vi "Respond.vi"(6 "String buffer in":string, 7 "String":string, 8 "error in (no error)":errorcluster, 9 "Return Request in":T1, 10 "Boolean in":bool, 11 "String 2":string) -> (0 "error out":errorcluster, 2 "String buffer out":string, 3 "Boolean out":bool)   [LabVIEW 2017, in "SSH.lvlib"]
uses:
  SSH.lvlib
  Return Request Configuration.ctl
  Response Configuration.ctl
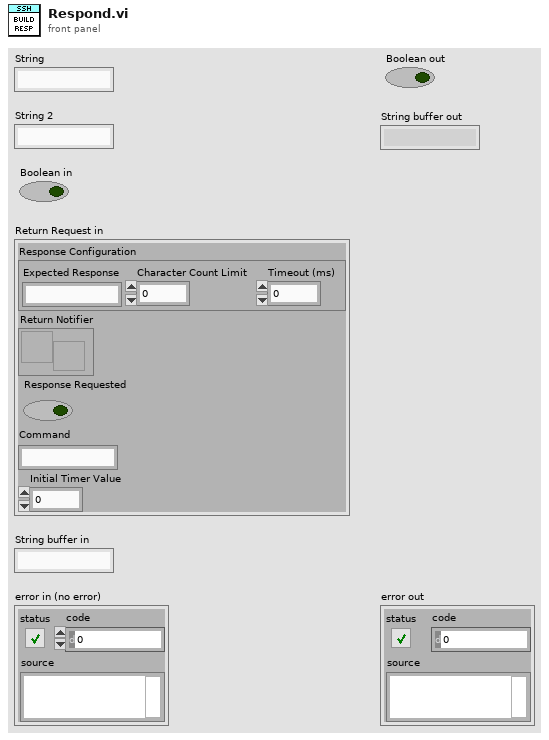
[diagram p1: front panel]
types:
  T1 = typedef "SSH.lvlib/Return Request Configuration.ctl" = cluster{"Response Configuration":T2, "Return Notifier":refnum<notifier>, "Response Requested":bool, "Command":string, "Initial Timer Value":u32}
  T2 = typedef "SSH.lvlib/Response Configuration.ctl" = cluster{"Expected Response":string, "Character Count Limit":i32, "Timeout (ms)":u32}
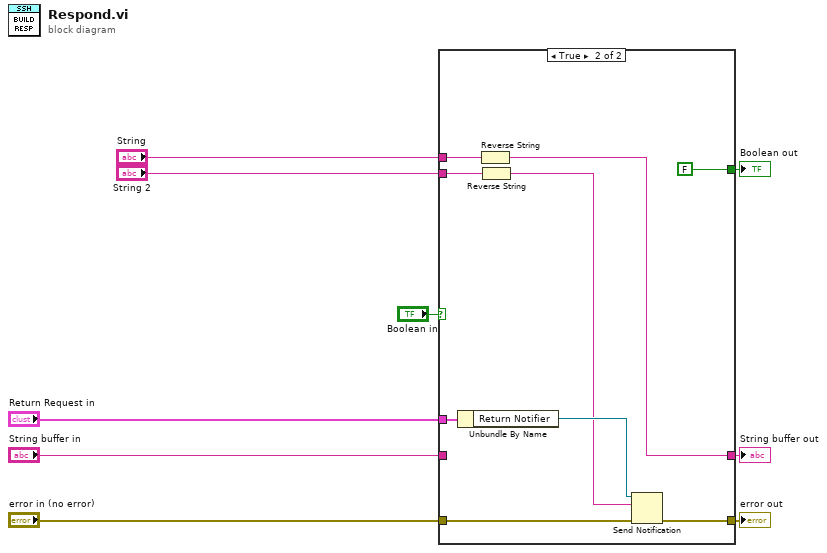
[diagram p0: block diagram]
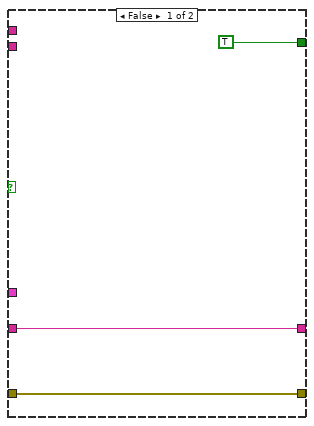
[diagram p2: hidden frame]
diagram:
  n1 = case shown="True" "Boolean in" {
    tunnel: [w10 w14] -> w1
    tunnel: "error in (no error)" -> [w11 w21]
    tunnel: [w11 w20] -> w3
    tunnel: "Return Request in" -> [_ w19]
    tunnel: [TRUE FALSE] -> w5
    tunnel: "String 2" -> [_ w15]
    tunnel: "String buffer in" -> [w10 _]
    tunnel: "String" -> [_ w16]
    frame False {
    }
    frame True {
      n2 = Unbundle By Name(w19) -> ("Return Notifier"=w18:refnum<notifier>)
      n3 = Reverse String(1:w16) -> (0:w14:string)
      n4 = Reverse String(1:w15) -> (0:w13:string)
      n5 = Send Notification(notification=w13, notifier=w18, error in (no error)=w21) -> (error out=w20:errorcluster)  [unwired: 1 out]
    }
  }
  "Boolean out" <- w5
  "error out" <- w3
  "String buffer out" <- w1
